vi "SMO.StartDependencies.vi"(8 "error in (no error)":errorcluster, 11 "SMO in":refnum<class "SMO.lvclass">) -> (0 "error out":errorcluster, 3 "SMO out":refnum<class "SMO.lvclass">)   [LabVIEW 2021, in "smo.lvlib" / "SMO.lvclass"]
uses:
  SMO.lvclass
  SMO.lvclass/SMO.ctl
  Dependency/Dependency.lvclass/Dependency.ctl
  ReftoDVR--SMO.vi
  Dependency/Dependency.lvclass
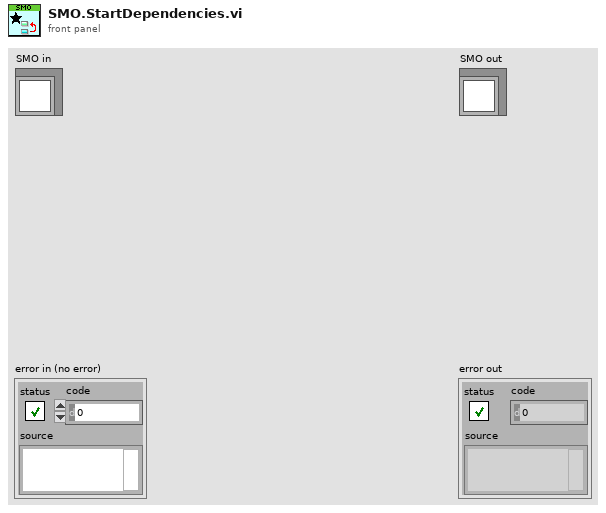
[diagram p1: front panel]
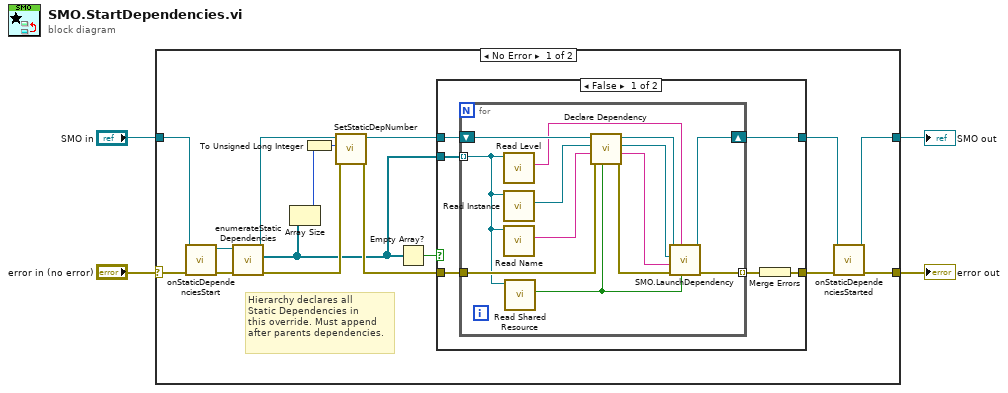
[diagram p0: block diagram]
diagram:
  n1 = case shown="No Error" "error in (no error)" {
    selector: "error in (no error)" -> [w12 w43]
    tunnel: [w9 w43] -> w2
    tunnel: [w7 w42] -> w3
    tunnel: "SMO in" -> [w5 w42]
    frame No Error {
      # "Hierarchy declares all\nStatic Dependencies in\nthis override. Must append\nafter parents dependencies."
      n2 = call-dynamic "onStaticDependenciesStart.vi"("error in (no error)"=w12, "SMO"=w5) -> ("error out"=w11:errorcluster, "SMO out"=w10:refnum<class "SMO.lvclass">)  [unwired: 8 in]
      n3 = call-dynamic "enumerateStaticDependencies.vi"("error in (no error)"=w11, "SMO"=w10) -> ("error out"=w19:errorcluster, "Static Dependencies"=w13:refnum<class "Dependency.lvclass">[], "SMO out"=w17:refnum<class "SMO.lvclass">)  [unwired: 7 in]
      n4 = Array Size(array=w13) -> (size(s)=w15:i32)
      n5 = To Unsigned Long Integer(number=w15) -> (unsigned 32bit integer=w14:u32)
      n6 = call "SetStaticDepNumber.vi"("error in (no error)"=w19, "Nb of Static Dependencies"=w14, "SMO in"=w17) -> ("error out"=w18:errorcluster, "SMO out"=w16:refnum<class "SMO.lvclass">)  [unwired: 7 in]
      n7 = Empty Array?(array=w13) -> (empty?=w20:bool)
      n8 = case shown="False" w20 {
        tunnel: w13 -> [w26 _]
        tunnel: w16 -> [w21 w41]
        tunnel: w18 -> [w24 w40]
        tunnel: [w23 w41] -> w6
        tunnel: [w22 w40] -> w8
        frame False {
          n9 = for {
            tunnel: w26 -> [w27] mode=indexing
            tunnel: w24 -> [w35]
            tunnel: [w39] -> w25 mode=indexing
            shift-right: [w38] -> w23
            shift-left: w21 -> [w37]
            n10 = call "Read Level.vi"("Dependency in"=w27) -> ("Level"=w28:string)  [unwired: 9 in, 1 out]
            n11 = call "Read Instance.vi"("Dependency in"=w27) -> ("SMO.lvclass"=w36:refnum<class "SMO.lvclass">)  [unwired: 9 in, 1 out]
            n12 = call "Read Name.vi"("Dependency in"=w27) -> ("Name"=w33:string)  [unwired: 9 in, 1 out]
            n13 = call "Read Shared Resource.vi"("Dependency in"=w27) -> ("Shared Resource"=w34:bool)  [unwired: 9 in, 1 out]
            n14 = call "Declare Dependency.vi"("Shared Resource"=w34, "error in (no error)"=w35, "Name"=w33, "Dependency"=w36, "SMO in"=w37) -> ("error out"=w29:errorcluster, "Unique Name"=w30:string, "Dependency out"=w31:refnum<class "SMO.lvclass">, "SMO out"=w32:refnum<class "SMO.lvclass">)  [unwired: 3 in]
            n15 = call "SMO.LaunchDependency.vi"("Shared Resource"=w34, "Level"=w28, "error in (no error)"=w29, "Dependency Name"=w30, "Dependency Type"=w31, "SMO in"=w32) -> ("error out"=w39:errorcluster, "SMO out"=w38:refnum<class "SMO.lvclass">)  [unwired: 2 in, 2 out]
          }
          n16 = Merge Errors(w25) -> (w22:errorcluster)
        }
        frame True {
        }
      }
      n17 = call-dynamic "onStaticDependenciesStarted.vi"("error in (no error)"=w8, "SMO"=w6) -> ("error out"=w9:errorcluster, "SMO out"=w7:refnum<class "SMO.lvclass">)  [unwired: 8 in]
    }
    frame Error {
    }
  }
  "error out" <- w2
  "SMO out" <- w3
